vi "AO_AI_Task_Multi.vi"(6 "OSC Configuration":T3(array[cluster])=[{"Signal Type"=enum."Sine Wave", "DC"=0.0, "Amplitude"=0.1, "frequency"=20.0, "Phase"=0.0}, {"Signal Type"=enum."Sine Wave", "DC"=0.0, "Amplitude"=0.19999999999999993, "frequency"=20.0, "Phase"=0.0}, {"Signal Type"=enum."Sine Wave", "DC"=0.0, "Amplitude"=0.30000000000000004, "frequency"=20.0, "Phase"=0.0}, {"Signal Type"=enum."Sine Wave", "DC"=0.0, "Amplitude"=0.4, "frequency"=20.0, "Phase"=0.0}] {"frequency" format="%0.2p"; "Amplitude" format="%0.2p"; "DC" format="%.2p"}, 7 "AO Configuration":T1(array[cluster])=[{"Output physical channels"="PXI1Slot2/ao0:1", "AO. Max"=10.0, "AO.Min"=-10.0}, {"Output physical channels"="PXI1Slot3/ao0:1", "AO. Max"=10.0, "AO.Min"=-10.0}], 8 "AI Configuration":T2(array[cluster])=[{"AI Rate"=200000.0, "AI Block Size"=20000, "AI Buffer Size (s)"=10, "AI.Coupling"=10050, "AI.Max"=10.0, "AI.Min"=-10.0, "Input physical channels"="PXI1Slot2/ai0:1"}, {"AI Rate"=200000.0, "AI Block Size"=20000, "AI Buffer Size (s)"=10, "AI.Coupling"=10050, "AI.Max"=10.0, "AI.Min"=-10.0, "Input physical channels"="PXI1Slot3/ai0:1"}] {"AI.Coupling" items=["AC"=10045, "DC"=10050, "GND"=10066]; "AI Rate" format="%.2f"}) -> (0 "Sampling information":cluster{"Fs":dbl, "#s":dbl}[](array[cluster])=[{"Fs"=200000.00004074536, "#s"=20000.0}], 1 "Actual AI rate":dbl[](array[numeric])=[200000.00004074536], 2 "AO Task":refnum<k21>[](array[refnum]), 3 "AI task":refnum<k21>[](array[refnum]))   [LabVIEW 2011]
uses:
  <vilib>/DAQmx/write.llb/DAQmx Write (Analog 1D Wfm NChan NSamp).vi
  <vilib>/DAQmx/create/channels.llb/DAQmx Create Channel (AI-Voltage-Basic).vi
  <vilib>/DAQmx/configure/timing.llb/DAQmx Timing (Sample Clock).vi
  <vilib>/DAQmx/create/channels.llb/DAQmx Create Channel (AO-Voltage-Basic).vi
  <vilib>/DAQmx/configure/trigger.llb/DAQmx Start Trigger (Digital Edge).vi
  <vilib>/DAQmx/miscellaneous.llb/DAQmx Fill In Error Info.vi
  C:/Program Files (x86)/National Instruments/LabVIEW 2011/resource/objmgr/daqmx.rc
  <vilib>/measure/NI_MABase.lvlib
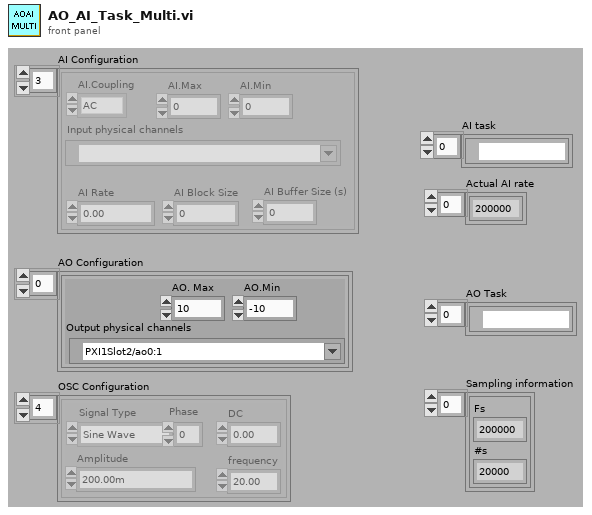
[diagram p1: front panel]
types:
  T1 = cluster{"Output physical channels":tag, "AO. Max":dbl, "AO.Min":dbl}[]
  T2 = cluster{"AI Rate":dbl, "AI Block Size":i32, "AI Buffer Size (s)":i32, "AI.Coupling":i32, "AI.Max":dbl, "AI.Min":dbl, "Input physical channels":tag}[]
  T3 = cluster{"Signal Type":enum16{"Sine Wave", "Triangle Wave", "Square Wave", "Sawtooth Wave"}, "DC":dbl, "Amplitude":dbl, "frequency":dbl, "Phase":dbl}[]
  T4 = enum16{"Sine Wave", "Triangle Wave", "Square Wave", "Sawtooth Wave"}
  T5 = cluster{"Signal Type":enum16{"Sine Wave", "Triangle Wave", "Square Wave", "Sawtooth Wave"}, "DC":dbl, "Amplitude":dbl, "frequency":dbl, "Phase":dbl}
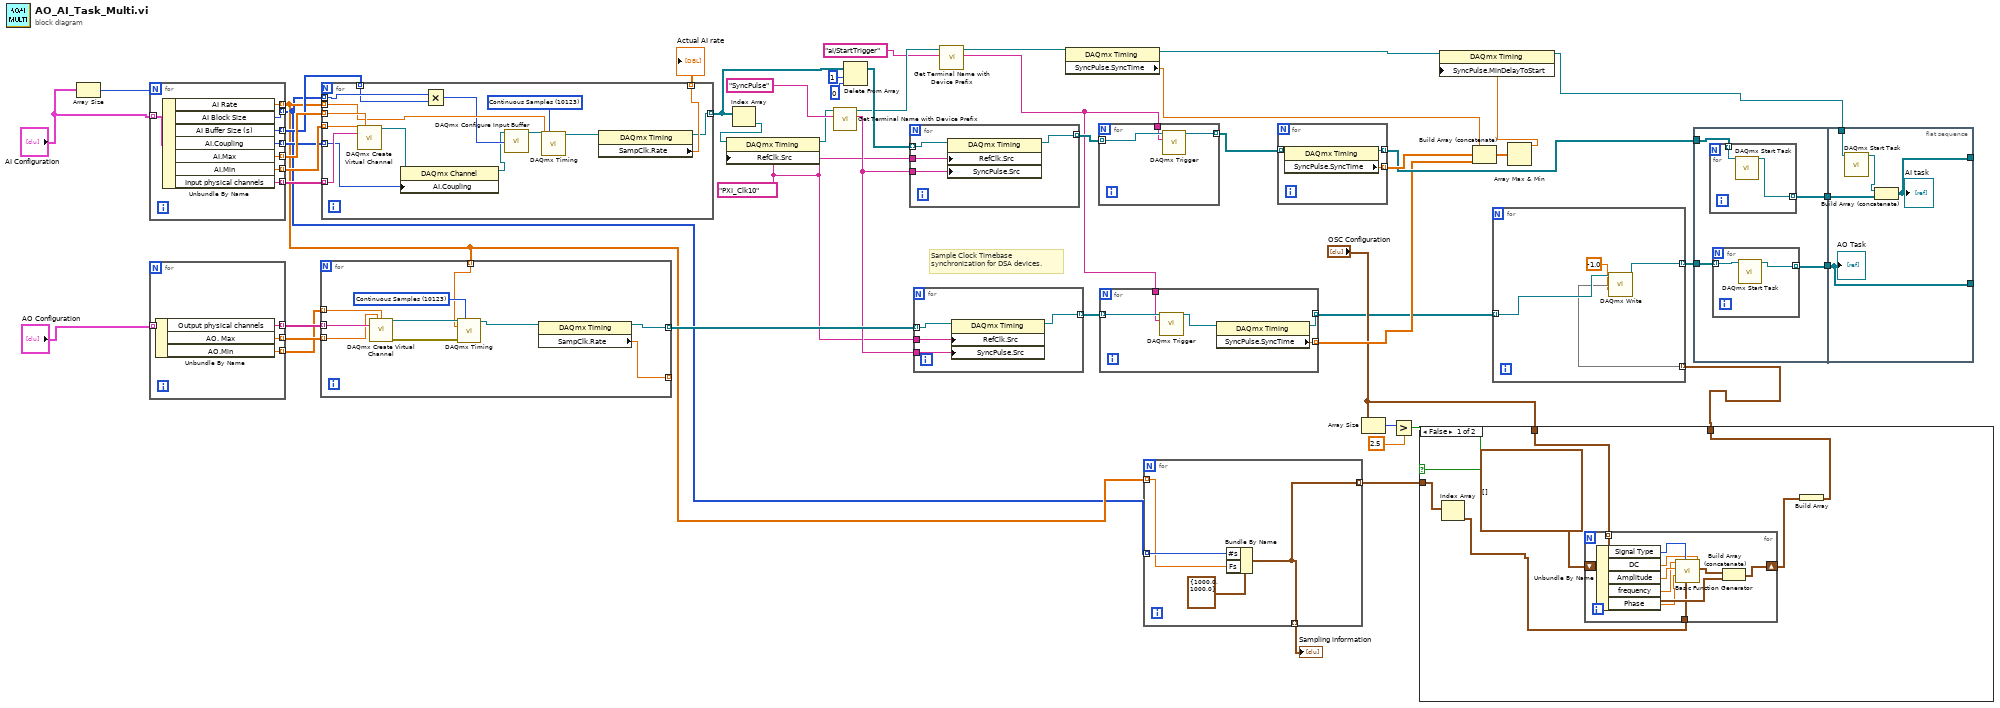
[diagram p0: block diagram]
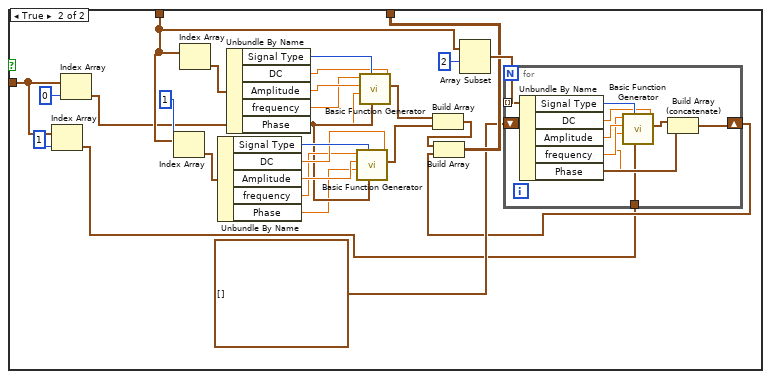
[diagram p2: hidden frame]
diagram:
  w11 = tag "PXI_Clk10" ("RefClk.Src")
  # "Sample Clock Timebase \nsynchronization for DSA devices."
  n1 = Array Size(array="AI Configuration") -> (size(s)=w50:i32)
  n2 = for {
    N: w50 -> [_]
    tunnel: "AI Configuration" -> [w58] mode=indexing
    tunnel: [w57] -> w40 mode=indexing
    tunnel: [w56] -> w48 mode=indexing
    tunnel: [w55] -> w47 mode=indexing
    tunnel: [w54] -> w4 mode=indexing
    tunnel: [w53] -> w3 mode=indexing
    tunnel: [w52] -> w42 mode=indexing
    tunnel: [w51] -> w16 mode=indexing
    n3 = Unbundle By Name(w58) -> ("AI Rate"=w54:dbl, "AI Block Size"=w53:i32, "AI Buffer Size (s)"=w52:i32, "AI.Coupling"=w51:i32, "AI.Max"=w55:dbl, "AI.Min"=w56:dbl, "Input physical channels"=w57:tag)
  }
  n4 = for {
    tunnel: "AO Configuration" -> [w62] mode=indexing
    tunnel: [w61] -> w45 mode=indexing
    tunnel: [w60] -> w44 mode=indexing
    tunnel: [w59] -> w43 mode=indexing
    n5 = Unbundle By Name(w62) -> ("Output physical channels"=w61:tag, "AO. Max"=w60:dbl, "AO.Min"=w59:dbl)
  }
  n6 = for {
    tunnel: w45 -> [w72] mode=indexing
    tunnel: w44 -> [w71] mode=indexing
    tunnel: w43 -> [w70] mode=indexing
    tunnel: [w66] -> w34 mode=indexing
    tunnel: [w65] -> _ mode=indexing
    tunnel: w4 -> [w63] mode=indexing
    w64 = 10123 items=["Finite Samples"=10178, "Continuous Samples"=10123, "Hardware Timed Single Point"=12522] ("sample mode")
    n7 = call-poly <vilib>:"DAQmx Create Virtual Channel.vi"("maximum value"=w71, "minimum value"=w70, "physical channels"=w72) -> ("task out"=w69:refnum<k21>, "error out"=w68:errorcluster)  [unwired: 11 in]
    n8 = call-poly <vilib>:"DAQmx Timing.vi"("task/channels in"=w69, "sample mode"=w64, "rate"=w63, "error in"=w68) -> ("task out"=w67:refnum<k21>)  [unwired: 10 in, 1 out]
    n9 = property class="DAQmx Timing"(reference=w67) -> (reference out=w66:refnum<k21>, "SampClk.Rate"=w65:dbl)  [unwired: 1 in, 1 out]
  }
  n10 = for {
    tunnel: w40 -> [w87] mode=indexing
    tunnel: w48 -> [w86] mode=indexing
    tunnel: w47 -> [w85] mode=indexing
    tunnel: w4 -> [w83] mode=indexing
    tunnel: w3 -> [w81] mode=indexing
    tunnel: w42 -> [w80] mode=indexing
    tunnel: [w77] -> w41 mode=indexing
    tunnel: [w76] -> w39 mode=indexing
    tunnel: w16 -> [w73] mode=indexing
    w84 = 10123 items=["Finite Samples"=10178, "Continuous Samples"=10123, "Hardware Timed Single Point"=12522] ("sample mode")
    n11 = call-poly <vilib>:"DAQmx Create Virtual Channel.vi"("maximum value"=w85, "minimum value"=w86, "physical channels"=w87) -> ("task out"=w75:refnum<k21>)  [unwired: 11 in, 1 out]
    n12 = property class="DAQmx Channel"(reference=w75, "AI.Coupling"=w73) -> (reference out=w74:refnum<k21>)  [unwired: 1 in, 1 out]
    n13 = Multiply(x=w81, y=w80) -> (x*y=w79:i32)
    n14 = call <vilib>:"DAQmx Configure Input Buffer.vi"("task/channels in"=w74, "buffer size (in samples per channel)"=w79) -> ("task out"=w82:refnum<k21>)  [unwired: 12 in, 1 out]
    n15 = call-poly <vilib>:"DAQmx Timing.vi"("task/channels in"=w82, "sample mode"=w84, "rate"=w83) -> ("task out"=w78:refnum<k21>)  [unwired: 11 in, 1 out]
    n16 = property class="DAQmx Timing"(reference=w78) -> (reference out=w76:refnum<k21>, "SampClk.Rate"=w77:dbl)  [unwired: 1 in, 1 out]
  }
  "Actual AI rate" <- w41
  n17 = Index Array(array=w39) -> (element=w13:refnum<k21>)  [unwired: 1 in]
  n18 = property class="DAQmx Timing"(reference=w13, "RefClk.Src"=w11) -> (reference out=w12:refnum<k21>)  [unwired: 1 in, 1 out]
  n19 = call "Get Terminal Name with Device Prefix.vi"("Local Terminal Name"="SyncPulse", "task/channels in"=w12) -> ("Terminal Name with Device Prefix"=w33:tag, "task out"=w31:refnum<k21>)  [unwired: 7 in, 1 out]
  n20 = Delete From Array(array=w39, length=1, index=0) -> (array with subset deleted=w35:refnum<k21>[])  [unwired: 1 out]
  n21 = for {
    tunnel: w35 -> [w91] mode=indexing
    tunnel: w11 -> [w90]
    tunnel: w33 -> [w89]
    tunnel: [w88] -> w32 mode=indexing
    n22 = property class="DAQmx Timing"(reference=w91, "RefClk.Src"=w90, "SyncPulse.Src"=w89) -> (reference out=w88:refnum<k21>)  [unwired: 1 in, 1 out]
  }
  n23 = for {
    tunnel: w34 -> [w95] mode=indexing
    tunnel: w11 -> [w94]
    tunnel: w33 -> [w93]
    tunnel: [w92] -> w29 mode=indexing
    n24 = property class="DAQmx Timing"(reference=w95, "RefClk.Src"=w94, "SyncPulse.Src"=w93) -> (reference out=w92:refnum<k21>)  [unwired: 1 in, 1 out]
  }
  n25 = call "Get Terminal Name with Device Prefix.vi"("Local Terminal Name"="ai/StartTrigger", "task/channels in"=w31) -> ("Terminal Name with Device Prefix"=w14:tag, "task out"=w28:refnum<k21>)  [unwired: 7 in, 1 out]
  n26 = property class="DAQmx Timing"(reference=w28) -> (reference out=w23:refnum<k21>, "SyncPulse.SyncTime"=w27:dbl)  [unwired: 1 in, 1 out]
  n27 = for {
    tunnel: w32 -> [w98] mode=indexing
    tunnel: w14 -> [w97]
    tunnel: [w96] -> w26 mode=indexing
    n28 = call-poly <vilib>:"DAQmx Trigger.vi"("task/channels in"=w98, "source"=w97) -> ("task out"=w96:refnum<k21>)  [unwired: 12 in, 1 out]
  }
  n29 = for {
    tunnel: w29 -> [w103] mode=indexing
    tunnel: [w101] -> w6 mode=indexing
    tunnel: [w100] -> w15 mode=indexing
    tunnel: w14 -> [w99]
    n30 = call-poly <vilib>:"DAQmx Trigger.vi"("task/channels in"=w103, "source"=w99) -> ("task out"=w102:refnum<k21>)  [unwired: 12 in, 1 out]
    n31 = property class="DAQmx Timing"(reference=w102) -> (reference out=w101:refnum<k21>, "SyncPulse.SyncTime"=w100:dbl)  [unwired: 1 in, 1 out]
  }
  n32 = for {
    tunnel: w4 -> [w106] mode=indexing
    tunnel: w3 -> [w107] mode=indexing
    tunnel: [w104] -> w2 mode=indexing
    tunnel: [w104] -> w1 mode=indexing
    n33 = Bundle By Name(cluster=cluster{"Fs":dbl, "#s":dbl} {"Fs"=1000.0, "#s"=1000.0} ("sampling info"), "#s"=w107, "Fs"=w106) -> (w104:cluster{"Fs":dbl, "#s":dbl})
  }
  "Sampling information" <- w2
  n34 = for {
    tunnel: w26 -> [w110] mode=indexing
    tunnel: [w109] -> w25 mode=indexing
    tunnel: [w108] -> w20 mode=indexing
    n35 = property class="DAQmx Timing"(reference=w110) -> (reference out=w108:refnum<k21>, "SyncPulse.SyncTime"=w109:dbl)  [unwired: 1 in, 1 out]
  }
  n36 = Array Size(array="OSC Configuration") -> (size(s)=w10:i32)
  n37 = Greater?(x=w10, y=2.5) -> (0:w8:bool)
  n38 = case shown="False" w8 {
    tunnel: "OSC Configuration" -> [w116 w140]
    tunnel: [w114 w137] -> w5
    tunnel: w1 -> [w112 w130]
    frame False {
      n39 = Index Array(array=w112) -> (element=w111:cluster{"Fs":dbl, "#s":dbl})  [unwired: 1 in]
      n40 = for {
        tunnel: w116 -> [w126] mode=indexing
        shift-right: [w119] -> w115
        shift-left: waveform(dbl)[] [] -> [w120]
        tunnel: w111 -> [w118]
        n41 = Unbundle By Name(w126) -> ("Signal Type"=w125:T4, "DC"=w124:dbl, "Amplitude"=w123:dbl, "frequency"=w122:dbl, "Phase"=w117:dbl)
        n42 = call <vilib>:"Basic Function Generator.vi"("offset"=w124, "sampling info"=w118, "signal type"=w125, "phase"=w117, "amplitude"=w123, "frequency"=w122) -> ("signal out"=w121:waveform(dbl))  [unwired: 3 in, 2 out]
        n43 = Build Array (concatenate)(w121, w120) -> (w119:waveform(dbl)[])
      }
      n44 = Build Array(w115) -> (w114:waveform(dbl)[][])
    }
    frame True {
      n45 = Index Array(array=w130, index=1) -> (element=w129:cluster{"Fs":dbl, "#s":dbl})
      n46 = Index Array(array=w130, index=0) -> (element=w131:cluster{"Fs":dbl, "#s":dbl})
      n47 = Index Array(array=w140, index=1) -> (element=w151:T5)
      n48 = Index Array(array=w140) -> (element=w152:T5)  [unwired: 1 in]
      n49 = Unbundle By Name(w151) -> ("Signal Type"=w146:T4, "DC"=w145:dbl, "Amplitude"=w144:dbl, "frequency"=w143:dbl, "Phase"=w127:dbl)
      n50 = Unbundle By Name(w152) -> ("Signal Type"=w150:T4, "DC"=w149:dbl, "Amplitude"=w148:dbl, "frequency"=w147:dbl, "Phase"=w128:dbl)
      n51 = call <vilib>:"Basic Function Generator.vi"("offset"=w145, "sampling info"=w131, "signal type"=w146, "phase"=w127, "amplitude"=w144, "frequency"=w143) -> ("signal out"=w141:waveform(dbl))  [unwired: 3 in, 2 out]
      n52 = call <vilib>:"Basic Function Generator.vi"("offset"=w149, "sampling info"=w131, "signal type"=w150, "phase"=w128, "amplitude"=w148, "frequency"=w147) -> ("signal out"=w142:waveform(dbl))  [unwired: 3 in, 2 out]
      n53 = Build Array(w142, w141) -> (w134:waveform(dbl)[])
      n54 = Array Subset(array=w140, index=2) -> (w138:T3)  [unwired: 1 in]
      n55 = for {
        tunnel: w138 -> [w163] mode=indexing
        shift-right: [w158] -> w135
        shift-left: waveform(dbl)[] [] -> [w157]
        tunnel: w129 -> [w155]
        n56 = Unbundle By Name(w163) -> ("Signal Type"=w162:T4, "DC"=w161:dbl, "Amplitude"=w160:dbl, "frequency"=w159:dbl, "Phase"=w154:dbl)
        n57 = call <vilib>:"Basic Function Generator.vi"("offset"=w161, "sampling info"=w155, "signal type"=w162, "phase"=w154, "amplitude"=w160, "frequency"=w159) -> ("signal out"=w156:waveform(dbl))  [unwired: 3 in, 2 out]
        n58 = Build Array (concatenate)(w156, w157) -> (w158:waveform(dbl)[])
      }
      n59 = Build Array(w134, w135) -> (w137:waveform(dbl)[][])
    }
  }
  n60 = Build Array (concatenate)(w27, w25, w15) -> (w24:dbl[])
  n61 = for {
    tunnel: w6 -> [w167] mode=indexing
    tunnel: [w166] -> w19 mode=indexing
    tunnel: w5 -> [w165] mode=indexing
    n62 = call-poly <vilib>:"DAQmx Write.vi"("task/channels in"=w167, "data"=w165, "timeout"=-1.0) -> ("task out"=w166:refnum<k21>)  [unwired: 10 in, 2 out]
  }
  n63 = Array Max & Min(array=w24) -> (max value=w22:dbl)  [unwired: 3 out]
  n64 = property class="DAQmx Timing"(reference=w23, "SyncPulse.MinDelayToStart"=w22) -> (reference out=w21:refnum<k21>)  [unwired: 1 in, 1 out]
  n65 = flat-sequence {
    tunnel: w20 -> [w171]
    tunnel: w19 -> [w170]
    tunnel: [w169] -> w18
    tunnel: [w168] -> w17
    tunnel: w21 -> [w180]
    tunnel: w18 -> [w178]
    tunnel: w17 -> [w176]
    tunnel: [w177] -> _
    tunnel: [w176] -> _
    frame #0 {
      n66 = for {
        tunnel: w171 -> [w175] mode=indexing
        tunnel: [w174] -> w169 mode=indexing
        n67 = call <vilib>:"DAQmx Start Task.vi"("task/channels in"=w175) -> ("task out"=w174:refnum<k21>)  [unwired: 13 in, 1 out]
      }
      n68 = for {
        tunnel: w170 -> [w173] mode=indexing
        tunnel: [w172] -> w168 mode=indexing
        n69 = call <vilib>:"DAQmx Start Task.vi"("task/channels in"=w173) -> ("task out"=w172:refnum<k21>)  [unwired: 13 in, 1 out]
      }
    }
    frame #1 {
      n70 = call <vilib>:"DAQmx Start Task.vi"("task/channels in"=w180) -> ("task out"=w179:refnum<k21>)  [unwired: 13 in, 1 out]
      n71 = Build Array (concatenate)(w179, w178) -> (w177:refnum<k21>[])
      "AI task" <- w177
      "AO Task" <- w176
    }
  }
